vi "GPIB FetchOF.vi"(3 "Bytes to Read":i16=200 step=10, 4 "Command String":string, 5 "GPIB Card":i16 min=0 max=3, 6 "GPIB Address":i16=15 max=30 step=1) -> (0 "Characters Read":string, 1 "Read Status":string, 2 "Write Status":string)   [LabVIEW 2023]
doc: "GPIB Fetch sends the Command String to the Addressed GPIB device, then reads the data back placing the results in Characters Read. Status strings are available for both read & write operations."
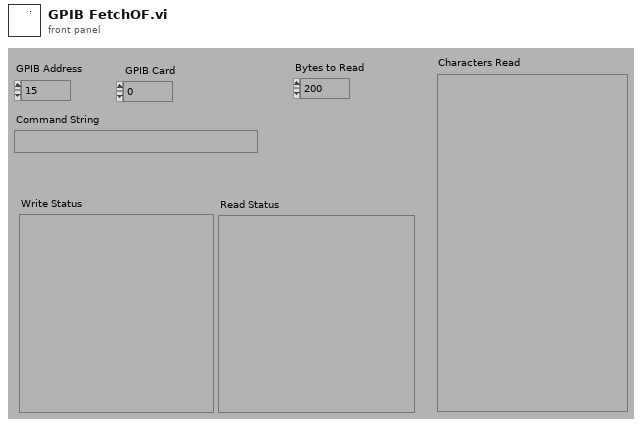
[diagram p1: front panel]
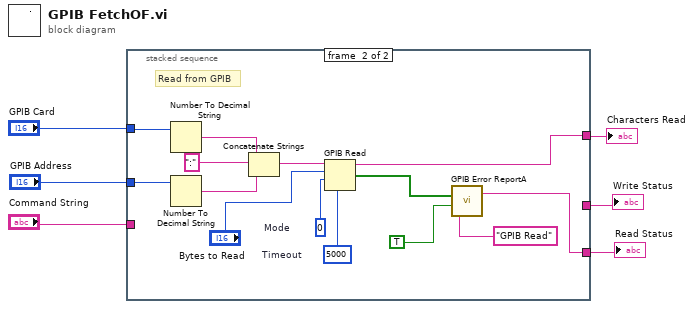
[diagram p0: block diagram]
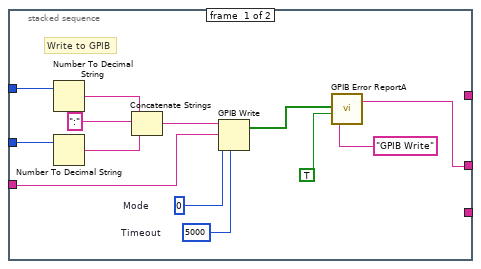
[diagram p2: hidden frame]
diagram:
  n1 = stacked-sequence {
    tunnel: "Command String" -> [w10 _]
    tunnel: [w15 _] -> w6
    tunnel: [_ w31] -> w5
    tunnel: "GPIB Card" -> [w17 w27]
    tunnel: "GPIB Address" -> [w16 w26]
    tunnel: [_ w21] -> w1
    frame #0 {
      w7 = u32 5000  # Timeout
      w8 = 0  # Mode
      # "Write to GPIB"
      n2 = Number To Decimal String(number=w17) -> (decimal integer string=w14:string)  [unwired: 1 in]
      n3 = Number To Decimal String(number=w16) -> (decimal integer string=w12:string)  [unwired: 1 in]
      n4 = Concatenate Strings(w14, ":", w12) -> (w11:string)
      n5 = GPIB Write(0:w11, 1:w10, 2:w8, 4:w7) -> (5:w9:bool[])  [unwired: 1 in, 1 out]
      n6 = call "GPIB Error ReportA.vi"("Function"="GPIB Write", "Dialog?(F)"=TRUE, "Status"=w9) -> ("Status String"=w15:string)  [unwired: 1 in, 1 out]
    }
    frame #1 {
      w22 = u32 5000  # Timeout
      w23 = 0  # Mode
      # "Read from GPIB"
      n7 = Number To Decimal String(number=w27) -> (decimal integer string=w30:string)  [unwired: 1 in]
      n8 = Number To Decimal String(number=w26) -> (decimal integer string=w28:string)  [unwired: 1 in]
      n9 = Concatenate Strings(w30, ":", w28) -> (w25:string)
      n10 = GPIB Read(0:w25, 1:"Bytes to Read", 2:w23, 4:w22) -> (5:w21:string, 6:w20:bool[])  [unwired: 1 in, 1 out]
      n11 = call "GPIB Error ReportA.vi"("Function"="GPIB Read", "Dialog?(F)"=TRUE, "Status"=w20) -> ("Status String"=w31:string)  [unwired: 1 in, 1 out]
    }
  }
  "Read Status" <- w5
  "Characters Read" <- w1
  "Write Status" <- w6
